vi "Apply Calibration.vi"(10 "Graph Data":waveform(dbl)[](array[waveform]), 11 "Calibration Array":T1[](array[typedef])) -> (2 "Calibrated Data":waveform(dbl)[](array[waveform]))   [LabVIEW 2024, in "Acquisition.lvlib"]
doc: "This VI applies the calibration constants to the data acquied.\n_____\nBased on DQMH Dev Tools: Project Template 7.1.0.1503."
uses:
  Acquisition.lvlib
  CML Shared/Calibration Values--cluster.ctl
  CML Shared/CML Shared.lvlib
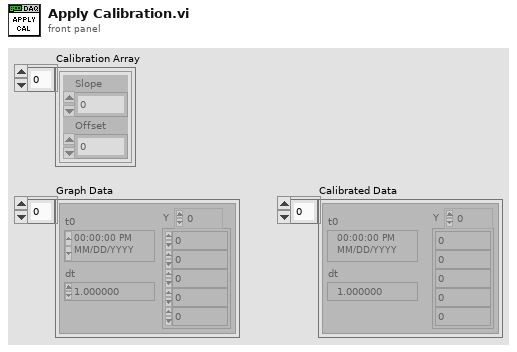
[diagram p1: front panel]
types:
  T1 = typedef "CML Shared.lvlib/Calibration Values--cluster.ctl" = cluster{"Slope":dbl, "Offset":dbl}
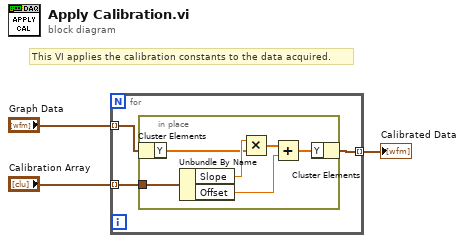
[diagram p0: block diagram]
diagram:
  # "This VI applies the calibration constants to the data acquired."
  n1 = for {
    tunnel: "Calibration Array" -> [w6] mode=indexing
    tunnel: "Graph Data" -> [w5] mode=indexing
    tunnel: [w4] -> w2 mode=indexing
    n2 = in-place "In Place Element Structure" {
      in-place-border: w6 -> [w12]
      n3 = in-place-cluster #1(w5) -> ("Y"=w7:dbl[])
      n4 = Unbundle By Name(w12) -> ("Slope"=w11:dbl, "Offset"=w9:dbl)
      n5 = Multiply(x=w11, y=w7) -> (x*y=w10:dbl[])
      n6 = Add(x=w10, y=w9) -> (x+y=w8:dbl[])
      n7 = in-place-cluster #1("Y"=w8) -> (w4:waveform(dbl))
    }
  }
  "Calibrated Data" <- w2
